vi "Reset Output Protection.vi"(8 "error in (no error)":errorcluster, 11 "VISA resource name":refnum<visa-resource-name>) -> (0 "error out":errorcluster, 3 "VISA resource name out":refnum<visa-resource-name>)   [LabVIEW 2018, in "XP Power PLS600.lvlib"]
doc: "Resets the status of over voltage protection (OVP), over current protection (OCP), and over power protection (OPP) by issuing an instrument reset command."
uses:
  XP Power PLS600.lvlib
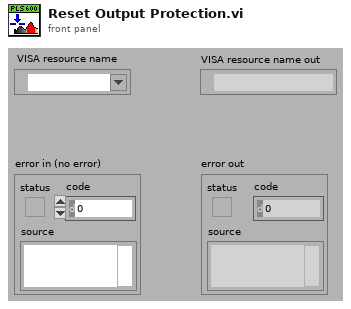
[diagram p1: front panel]
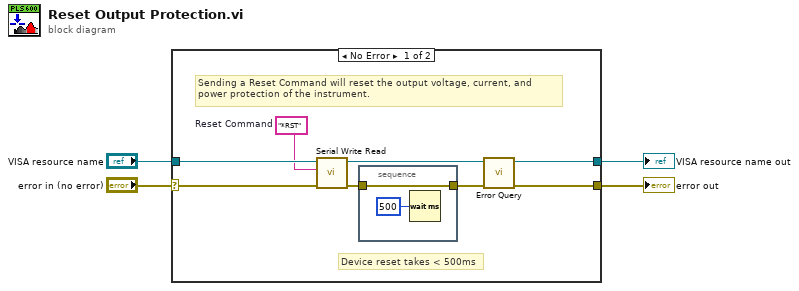
[diagram p0: block diagram]
diagram:
  n1 = case shown="No Error" "error in (no error)" {
    selector: "error in (no error)" -> [w5 w16]
    tunnel: [w12 w15] -> w4
    tunnel: [w11 w16] -> w3
    tunnel: "VISA resource name" -> [w9 w15]
    frame No Error {
      w8 = "*RST"  # Reset Command
      # "Device reset takes < 500ms"
      # "Sending a Reset Command will reset the output voltage, current, and\npower protection of the instrument."
      n2 = call "Serial Write Read.vi"("error in (no error)"=w5, "Write Buffer"=w8, "VISA resource name"=w9) -> ("error out"=w6:errorcluster, "VISA resource name out"=w7:refnum<visa-resource-name>)  [unwired: 6 in, 1 out]
      n3 = stacked-sequence {
        tunnel: w6 -> [w14]
        tunnel: [w14] -> w10
        frame #0 {
          n4 = Wait (ms)(milliseconds to wait=u32 500) -> ()  [unwired: 1 out]
        }
      }
      n5 = call "Error Query.vi"("error in (no error)"=w10, "VISA resource name"=w7) -> ("error out"=w11:errorcluster, "VISA resource name out"=w12:refnum<visa-resource-name>)  [unwired: 6 in, 2 out]
    }
    frame Error {
    }
  }
  "VISA resource name out" <- w4
  "error out" <- w3
